vi "DiffDriveVoltageConstraint_New.vi"(9 "SIMPLE_MOTOR_FF":T1 {"Ka" format="%13.4f"; "Kv" format="%13.4f"; "Ks" format="%13.4f"}, 10 "DIFF_DRIVE_KINEMATICS":T2 {"TrackWidth_Meters" format="%20.4f"}, 11 "Max Voltage":dbl format="%20.4f") -> (3 "DIFF_DRIVE_VOLTAGE_CONSTRAINT":T3 {"SIMPLE_MOTOR_FF"."Ka" format="%13.4f"; "SIMPLE_MOTOR_FF"."Kv" format="%13.4f"; "SIMPLE_MOTOR_FF"."Ks" format="%13.4f"; "DIFF_DRIVE_KINEMATICS"."TrackWidth_Meters" format="%20.4f"; "Max Voltage" format="%20.4f"})   [LabVIEW 2019, in "Trajectory_Library.lvlib"]
doc: "Creates a new DifferentialDriveVoltageConstraint.\n\nParameters:\n - maxVoltage - The maximum voltage available to the motors while following the path. Should be somewhat less than the nominal battery voltage (12V) to account for \"voltage sag\" due to current draw.\n - DiffDriveKinematics - A kinematics component describing the drive geometry.\n - SimpleMotorFeedforward - A feedforward component describing the behavior of the drive.\n\nReturns\n - DiffDriveVoltageConstraint - Constraint data structure"
uses:
  Trajectory_Library.lvlib
  TypeDef/TRAJ_CONSTRAINT_DIIF_DRIVE_VOLTAGE.ctl
  TypeDef/DIFF_DRIVE_KINEMATICS.ctl
  TypeDef/SIMPLE_MOTOR_FF.ctl
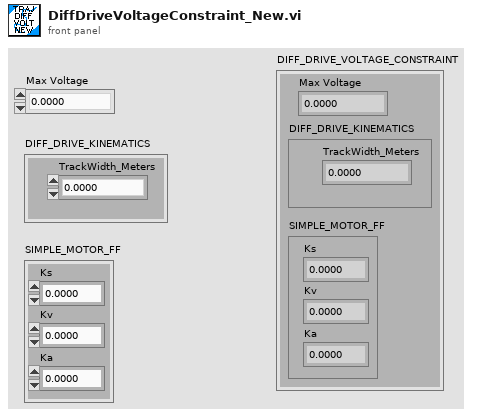
[diagram p1: front panel]
types:
  T1 = typedef "Trajectory_Library.lvlib/SIMPLE_MOTOR_FF.ctl" = cluster{"Ks":dbl, "Kv":dbl, "Ka":dbl}
  T2 = typedef "Trajectory_Library.lvlib/DIFF_DRIVE_KINEMATICS.ctl" = cluster{"TrackWidth_Meters":dbl}
  T3 = typedef "Trajectory_Library.lvlib/TRAJ_CONSTRAINT_DIIF_DRIVE_VOLTAGE.ctl" = cluster{"Max Voltage":dbl, "DIFF_DRIVE_KINEMATICS":T2, "SIMPLE_MOTOR_FF":T1}
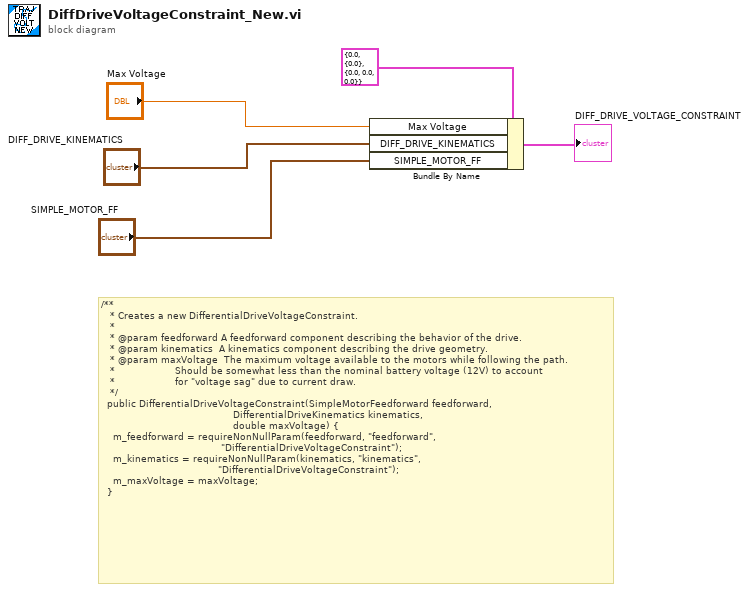
[diagram p0: block diagram]
diagram:
  # "/**\n   * Creates a new DifferentialDriveVoltageConstraint.\n   *\n   * @param feedforward A feedforward component describing the behavior of the drive.\n   * @param kinematics  A kinematics component describing the drive geometry.\n   * @param maxVoltage  The maximum voltage available to the motors while following the path.\n   *                    Should be somewhat less than the nominal battery voltage (12V) to account\n   *                    for \"voltage sag\" due to current draw.\n   */\n  public DifferentialDriveVoltageConstraint(SimpleMotorFeedforward feedforward,\n                                            DifferentialDriveKinematics kinematics,\n                                            double maxVoltage) {\n    m_feedforward = requireNonNullParam(feedforward, \"feedforward\",\n                                        \"DifferentialDriveVoltageConstraint\");\n    m_kinematics = requireNonNullParam(kinematics, \"kinematics\",\n                                       \"DifferentialDriveVoltageConstraint\");\n    m_maxVoltage = maxVoltage;\n  }"
  n1 = Bundle By Name(cluster=T3 {"Max Voltage"=0.0, "DIFF_DRIVE_KINEMATICS"={"TrackWidth_Meters"=0.0}, "SIMPLE_MOTOR_FF"={"Ks"=0.0, "Kv"=0.0, "Ka"=0.0}} ("DIFF_DRIVE_VOLTAGE_CONSTRAINT"), "Max Voltage"="Max Voltage", "DIFF_DRIVE_KINEMATICS"="DIFF_DRIVE_KINEMATICS", "SIMPLE_MOTOR_FF"="SIMPLE_MOTOR_FF") -> (→"DIFF_DRIVE_VOLTAGE_CONSTRAINT":T3)
